vi "Manually Remove Actor.vi"(8 "error in (no error)":errorcluster, 10 "Actor's Q":refnum<class "Message Enqueuer.lvclass">, 11 "Actor Monitor New in":refnum<class "Actor Monitor.lvclass">) -> (0 "error out":errorcluster, 3 "Actor Monitor New out":refnum<class "Actor Monitor.lvclass">)   [LabVIEW 2017, in "MGI-Monitored Actor Core.lvlib" / "Actor Monitor.lvclass"]
doc: "Removes the actor from the monitoring list\n\nCopyright: MGI 2016\nAuthor: Derek Trepanier"
uses:
  Actor Monitor.lvclass
  <vilib>/ActorFramework/Message Enqueuer/Message Enqueuer.lvclass
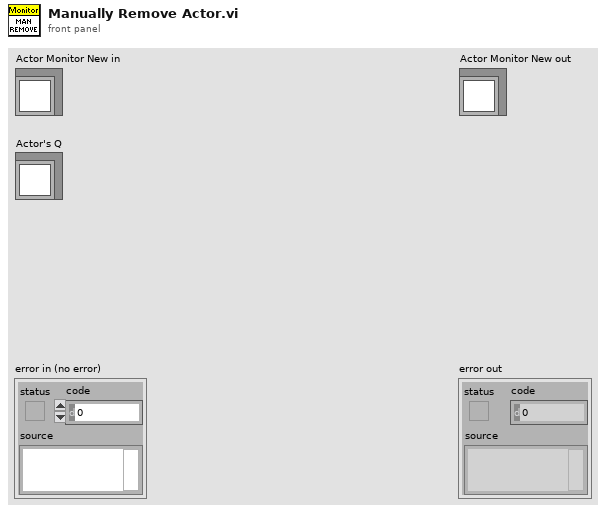
[diagram p1: front panel]
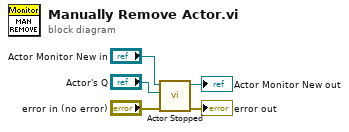
[diagram p0: block diagram]
diagram:
  n1 = call "Actor Stopped.vi"("error in (no error)"="error in (no error)", "Actor's Self Q"="Actor's Q", "Actor Monitor New in"="Actor Monitor New in") -> ("error out"=→"error out":errorcluster, "Actor Monitor New out"=→"Actor Monitor New out":refnum<class "Actor Monitor.lvclass">)  [unwired: 7 in]
